vi "PID_reg.vi"() -> ()   [LabVIEW 2017]
panel:
  out "String":string
  in  "stop":bool
  in  "Knob":dbl(knob) scale=0.0..10.0
  out "Gauge":dbl(knob) scale=0.0..6000.0
  in  "IP address":string
  in  "remote port\n or service name":u16
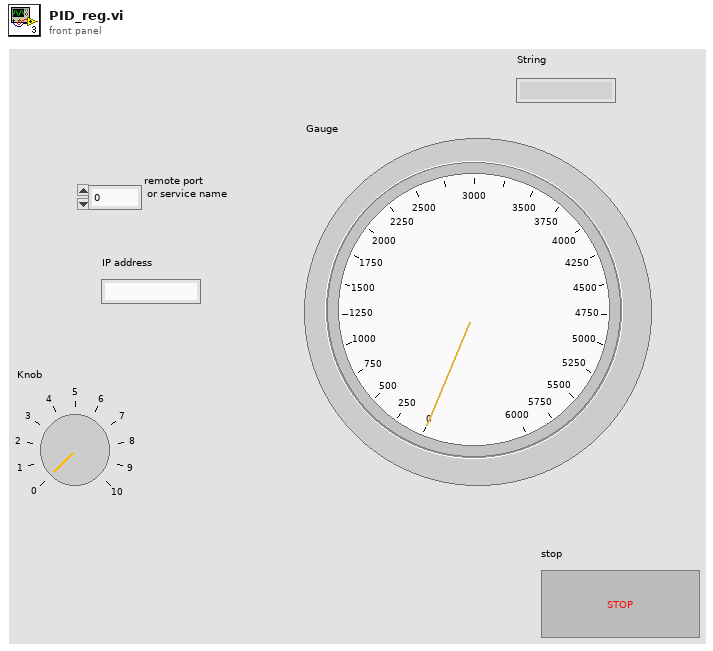
[diagram p1: front panel]
types:
  T1 = enum16{"Standard", "Buffered", "CRLF", "Immediate"}
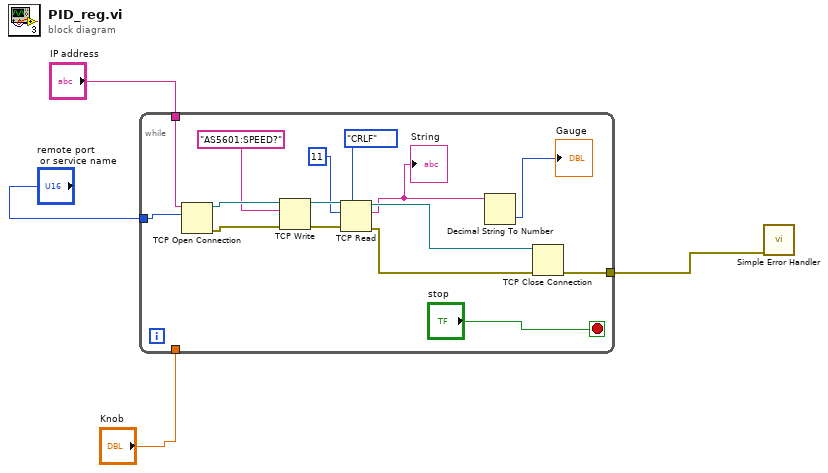
[diagram p0: block diagram]
diagram:
  n1 = while {
    tunnel: "Knob" -> [_]
    tunnel: "remote port\n or service name" -> [w15]
    tunnel: "IP address" -> [w14]
    tunnel: [w9] -> w2
    stop <- "stop" stop-if-true
    n2 = TCP Open Connection(address=w14, remote port or service name=w15) -> (connection ID=w12:refnum<k5>, error out=w13:errorcluster)  [unwired: 3 in]
    n3 = TCP Write(connection ID=w12, data in="AS5601:SPEED?", error in (no error)=w13) -> (connection ID out=w19:refnum<k5>, error out=w16:errorcluster)  [unwired: 1 in, 1 out]
    n4 = TCP Read(connection ID=w19, bytes to read=11, error in (no error)=w16, 7:T1."CRLF" ("mode (standard)")) -> (connection ID out=w10:refnum<k5>, data out=w7:string, error out=w11:errorcluster)  [unwired: 1 in]
    "String" <- w7
    n5 = Decimal String To Number(string=w7) -> (number=→"Gauge":i32)  [unwired: 2 in, 1 out]
    n6 = TCP Close Connection(connection ID=w10, error in (no error)=w11) -> (error out=w9:errorcluster)  [unwired: 1 in, 1 out]
  }
  n7 = call <vilib>:"Simple Error Handler.vi"("error in (no error)"=w2) -> ()  [unwired: 4 in, 5 out]
